vi "Exit.vi"(8 "error in (no error)":errorcluster, 11 "CI Mediator in":refnum<class "CI Mediator.lvclass">) -> (0 "error out":errorcluster, 3 "CI Mediator out":refnum<class "CI Mediator.lvclass">)   [LabVIEW 2014, in "CI Mediator.lvlib" / "CI Mediator.lvclass"]
uses:
  CI Mediator.lvclass
  CI Mediator.lvclass/CI Mediator.ctl
  <vilib>/ActorFramework/Actor/Actor.lvclass/Actor.ctl
  <vilib>/ActorFramework/Message Enqueuer/Message Enqueuer.lvclass/Message Enqueuer.ctl
  <vilib>/ActorFramework/Message Enqueuer/Init from Existing Queue.vi
  <vilib>/ActorFramework/Message Enqueuer/Enqueue.vi
  <vilib>/ActorFramework/Message Priority Queue/Priority Enqueue.vi
  <vilib>/ActorFramework/Message Enqueuer/Message Enqueuer.lvclass
  <vilib>/ActorFramework/Stop Msg/Stop Msg.lvclass
  Classes/Executor/Executor.lvclass
  <vilib>/ActorFramework/Actor/Actor.lvclass
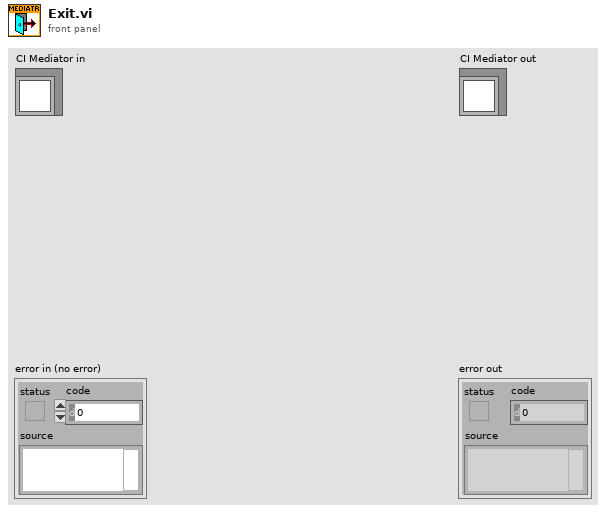
[diagram p1: front panel]
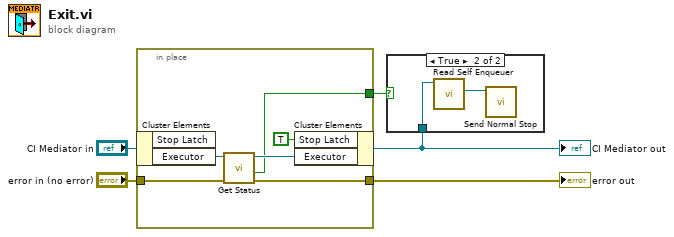
[diagram p0: block diagram]
diagram:
  n1 = in-place {
    in-place-border: "error in (no error)" -> [w9]
    in-place-border: [w8] -> w3
    in-place-border: [w6] -> w1
    n2 = in-place-cluster #1("CI Mediator in") -> ("Executor"=w11:refnum<class "Executor.lvclass">)  [unwired: 1 out]
    n3 = call "Get Status.vi"("error in (no error)"=w9, "Executor Reference"=w11) -> ("error out"=w8:errorcluster, "Safe Shutdown?"=w6:bool, "Executor Reference"=w10:refnum<class "Executor.lvclass">)  [unwired: 6 in, 1 out]
    n4 = in-place-cluster #1("Stop Latch"=TRUE, "Executor"=w10) -> (w2:refnum<class "CI Mediator.lvclass">)
  }
  "error out" <- w3
  "CI Mediator out" <- w2
  n5 = case shown="True" w1 {
    tunnel: w2 -> [_ w13]
    frame False {
    }
    frame True {
      n6 = call <vilib>:"Read Self Enqueuer.vi"("Actor"=w13) -> ("Self Enqueuer"=w12:refnum<class "Message Enqueuer.lvclass">)  [unwired: 10 in]
      n7 = call <vilib>:"Send Normal Stop.vi"("Message Enqueuer"=w12) -> ()  [unwired: 10 in, 1 out]
    }
  }
